vi "Retrieve Scaling and Convert AI to EngUnits.vi"(7 "bypass (F)":bool, 8 "error in (no error)":errorcluster, 9 "RawValue in":dbl, 10 "IOName":string, 11 "DAQ Node Dict DVR":T1) -> (0 "error out":errorcluster, 1 "Engineering Units Out":dbl, 2 "IOName out":string, 3 "DAQ Node Dict DVR out":T1)   [LabVIEW 2017, in "DAQ.lvclass"]
doc: "Developed by Kevin Thompson\nkevin@thompsonengineering.net\n\nCopyright 2018-2020\nThompson Engineering, LLC"
uses:
  DAQ.lvclass
  <vilib>/TELLC/Dynamic CVT API/TD Dynamic CVT DVR--ref.ctl
  DataTypes/TD AI Channel--cluster.ctl
  DataTypes/TD DataValueConversion--cluster.ctl
  DataTypes/TD AI DAQ Type--enum.ctl
  DataTypes/TD AI Force Bridge--cluster.ctl
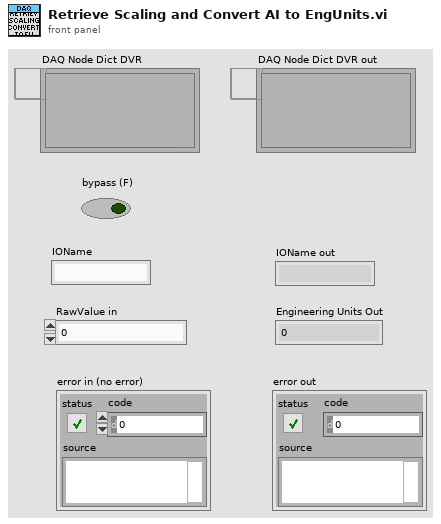
[diagram p1: front panel]
types:
  T1 = typedef "TD Dynamic CVT DVR--ref.ctl" = refnum<data-value>
  T2 = typedef "DAQ.lvclass/TD AI Channel--cluster.ctl" = cluster{"DevName":string, "IOName":string, "IOPath":string, "SchemName":string, "MinValue":dbl, "MaxValue":dbl, "Terminal Configuration":i32, "Index":i32, "Conversion":T3, "AIType":T4, "Force Bridge":T5}
  T3 = typedef "DAQ.lvclass/TD DataValueConversion--cluster.ctl" = cluster{"MaxSignal":dbl, "MinSignal":dbl, "MaxEngUnit":dbl, "MinEngUnit":dbl, "ScaleOffset":dbl, "negate":bool}
  T4 = typedef "DAQ.lvclass/TD AI DAQ Type--enum.ctl" = enum16{"Voltage", "Current", "Strain Gage", "Force Bridge"}
  T5 = typedef "DAQ.lvclass/TD AI Force Bridge--cluster.ctl" = cluster{"bridge information":cluster{"bridge configuration":i32, "voltage excitation source":i32, "voltage excitation value":dbl, "nominal bridge resistance":dbl}, "scaling information":cluster{"first electrical value":dbl, "second electrical value":dbl, "electrical units":i32, "first physical value":dbl, "second physical value":dbl, "physical units":i32}}
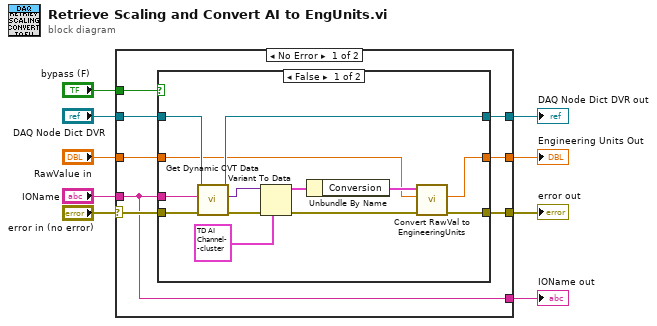
[diagram p0: block diagram]
diagram:
  n1 = case shown="No Error" "error in (no error)" {
    selector: "error in (no error)" -> [w12 w36]
    tunnel: [w17 w35] -> w9
    tunnel: [w16 w36] -> w8
    tunnel: "IOName" -> [w10 w34]
    tunnel: "DAQ Node Dict DVR" -> [w15 w37]
    tunnel: [w14 w37] -> w5
    tunnel: "RawValue in" -> [w13 w35]
    tunnel: "bypass (F)" -> [w11 _]
    tunnel: [w10 w34] -> w1
    frame No Error {
      n2 = case shown="False" w11 {
        tunnel: [w30 w32] -> w17
        tunnel: [w29 w31] -> w16
        tunnel: w10 -> [w23 _]
        tunnel: w15 -> [w22 w33]
        tunnel: [w21 w33] -> w14
        tunnel: w13 -> [w20 w32]
        tunnel: w12 -> [w19 w31]
        frame False {
          n3 = call <vilib>:"Get Dynamic CVT Data.vi"("error in (no error)"=w19, "DataName"=w23, "dCVT DVR"=w22) -> ("error out"=w25:errorcluster, "value"=w24:variant, "dCVT DVR out"=w21:T1)  [unwired: 5 in, 1 out]
          n4 = Variant To Data(error in=w25, type=T2 {"DevName"="", "IOName"="", "IOPath"="", "SchemName"="", "MinValue"=0.0, "MaxValue"=0.0, "Terminal Configuration"=0, "Index"=0, "Conversion"={"MaxSignal"=0.0, "MinSignal"=0.0, "MaxEngUnit"=0.0, "MinEngUnit"=0.0, "ScaleOffset"=0.0, "negate"=FALSE}, "AIType"=enum."Voltage", "Force Bridge"={"bridge information"={"bridge configuration"=10182, "voltage excitation source"=10200, "voltage excitation value"=2.5, "nominal bridge resistance"=350.0}, "scaling information"={"first electrical value"=0.0, "second electrical value"=2.0, "electrical units"=15897, "first physical value"=0.0, "second physical value"=100.0, "physical units"=15876}}} ("AI"), Variant=w24) -> (data=w26:T2, error out=w28:errorcluster)
          n5 = Unbundle By Name(w26) -> ("Conversion"=w27:T3)
          n6 = call "Convert RawVal to EngineeringUnits.vi"("error in (no error)"=w28, "Raw Value In"=w20, "Conversion"=w27) -> ("error out"=w29:errorcluster, "Engineering Units Out"=w30:dbl)  [unwired: 7 in]
        }
        frame True {
        }
      }
    }
    frame Error {
    }
  }
  "Engineering Units Out" <- w9
  "error out" <- w8
  "DAQ Node Dict DVR out" <- w5
  "IOName out" <- w1
